vi "readAvailable.vi"(8 "error in (no error)":errorcluster, 11 "SerialReal in":refnum<class "SerialReal.lvclass">) -> (0 "error out":errorcluster, 2 "stringRead":string, 3 "SerialReal out":refnum<class "SerialReal.lvclass">)   [LabVIEW 2015, in "SerialProtocols.lvlib" / "SerialReal.lvclass"]
uses:
  <userlib>/Common/SerialProtocols/SerialProtocol/SerialReal/SerialReal.lvclass
  <userlib>/Common/SerialProtocols/SerialProtocol/SerialReal/SerialReal.lvclass/SerialReal.ctl
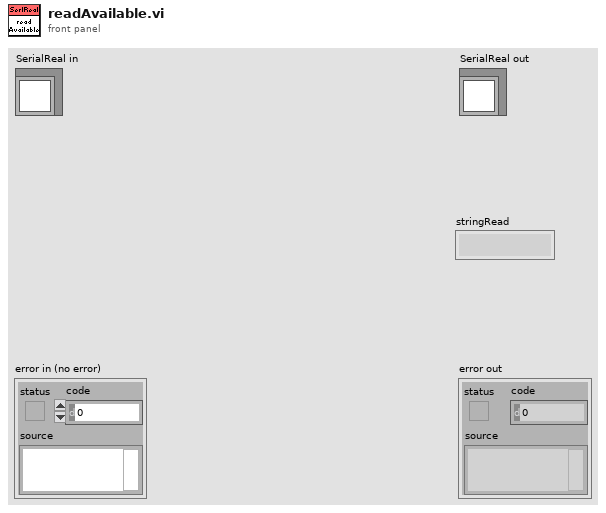
[diagram p1: front panel]
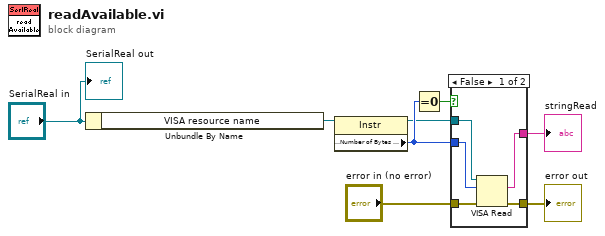
[diagram p0: block diagram]
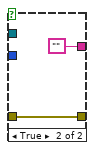
[diagram p2: hidden frame]
diagram:
  n1 = Unbundle By Name("SerialReal in") -> ("VISA resource name"=w8:refnum<visa-resource-name>)
  n2 = property class="Instr"(reference=w8) -> (reference out=w5:refnum<visa-resource-name>, "Serial Settings:Number of Bytes at Serial Port"=w6:u32)  [unwired: 1 in, 1 out]
  n3 = Equal To 0?(x=w6) -> (x = 0?=w7:bool)
  n4 = case shown="False" w7 {
    tunnel: w6 -> [w13 _]
    tunnel: w5 -> [w12 _]
    tunnel: [w11 ""] -> w4
    tunnel: "error in (no error)" -> [w10 w15]
    tunnel: [w9 w15] -> w2
    frame False {
      n5 = VISA Read(VISA resource name=w12, byte count=w13, error in (no error)=w10) -> (read buffer=w11:string, error out=w9:errorcluster)  [unwired: 2 out]
    }
    frame True {
    }
  }
  "error out" <- w2
  "stringRead" <- w4
  "SerialReal out" <- "SerialReal in"
